vi "Update Bind RPC Template.vi"(8 "error in (no error)":errorcluster, 11 "Server Library (Library Item) in":refnum<vi>) -> (0 "error out":errorcluster, 3 "Server Library (Library Item) out":refnum<vi>)   [LabVIEW 2019, in "gRPC Scripting Tools.lvlib"]
uses:
  gRPC Scripting Tools.lvlib
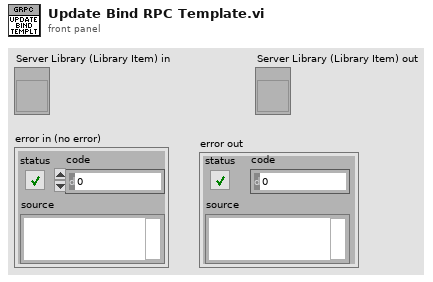
[diagram p1: front panel]
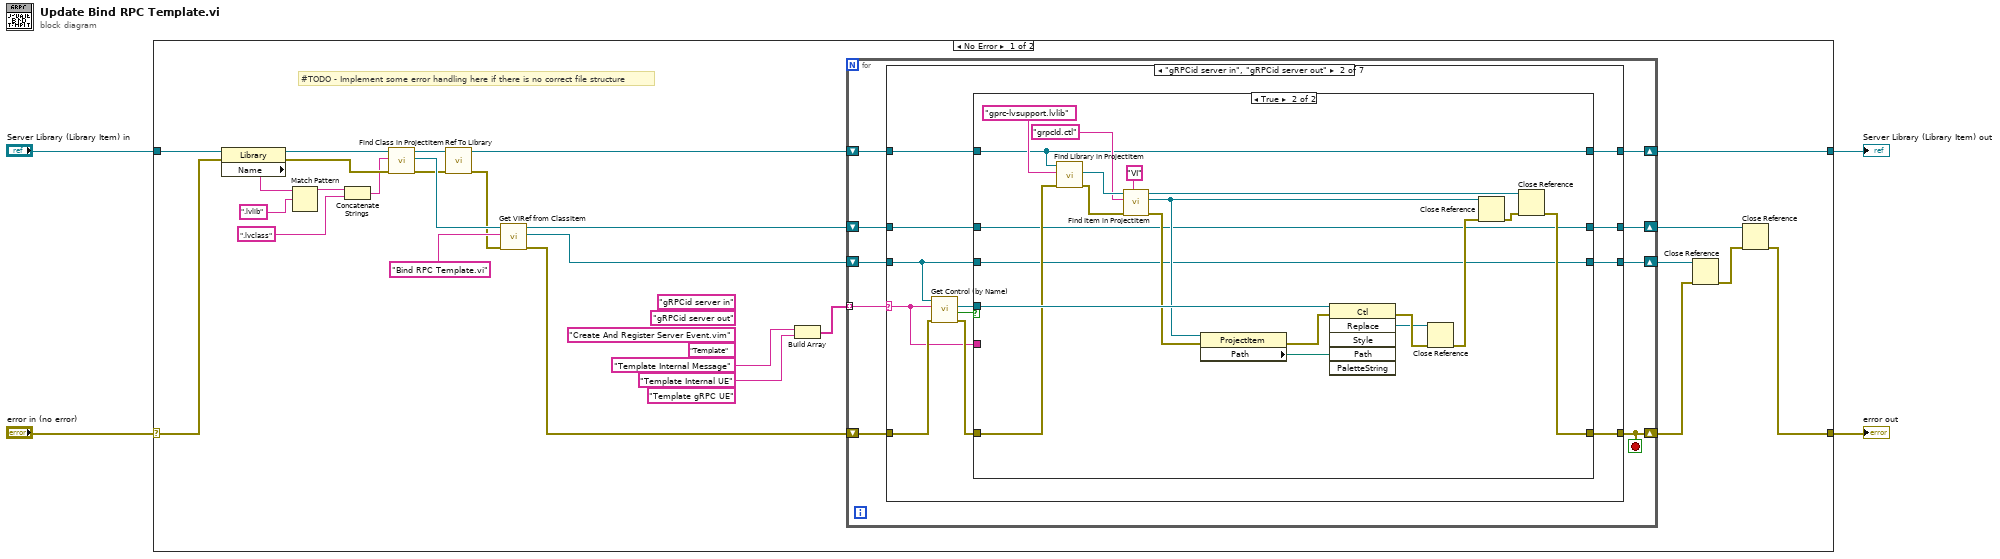
[diagram p0: block diagram]
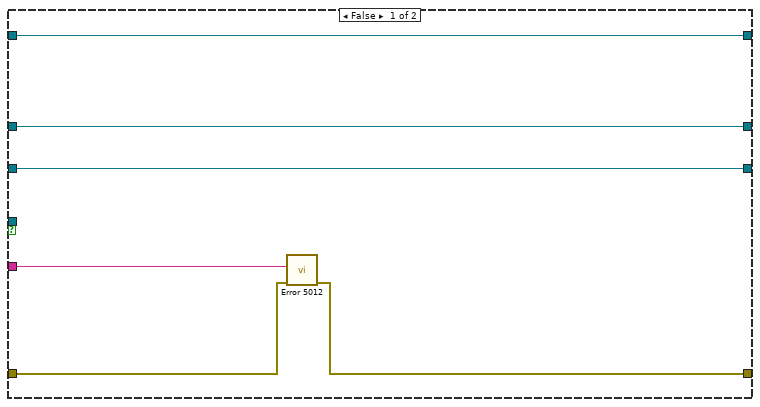
[diagram p3: hidden frame]
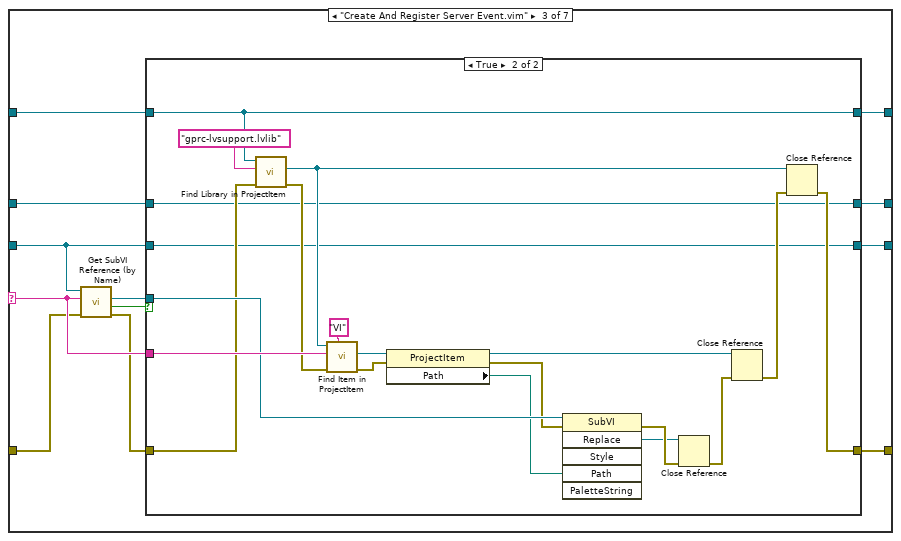
[diagram p4: hidden frame]
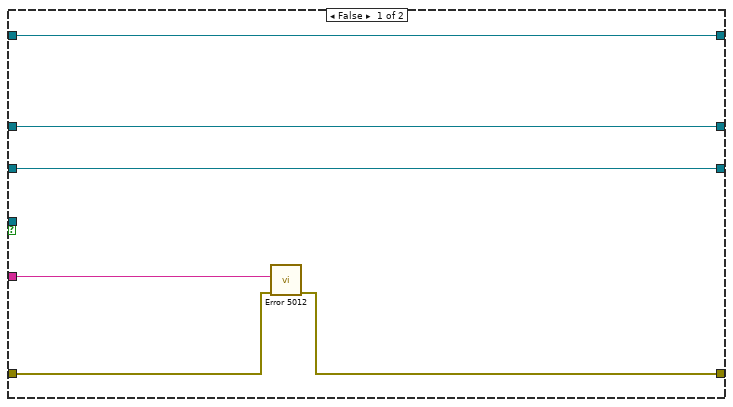
[diagram p5: hidden frame]
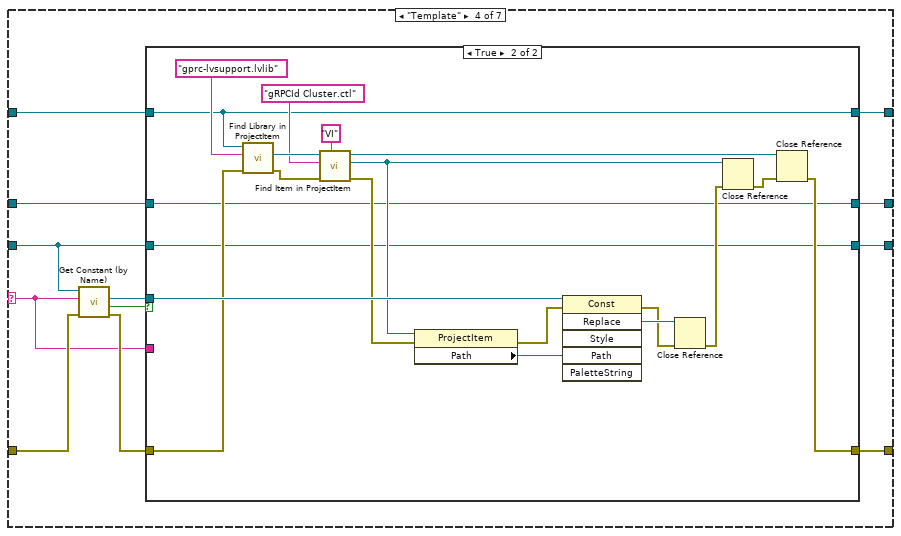
[diagram p6: hidden frame]
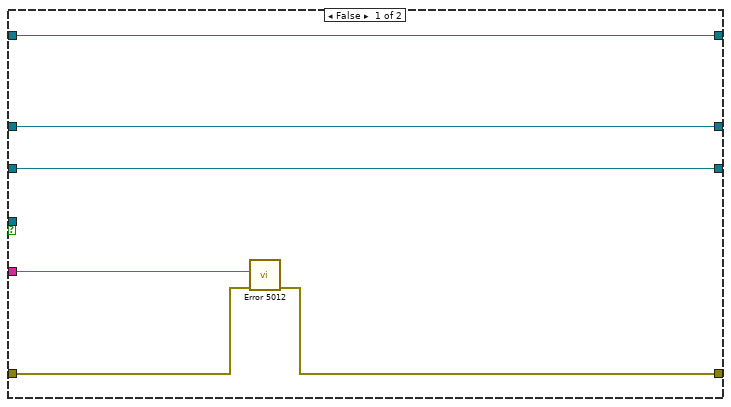
[diagram p7: hidden frame]
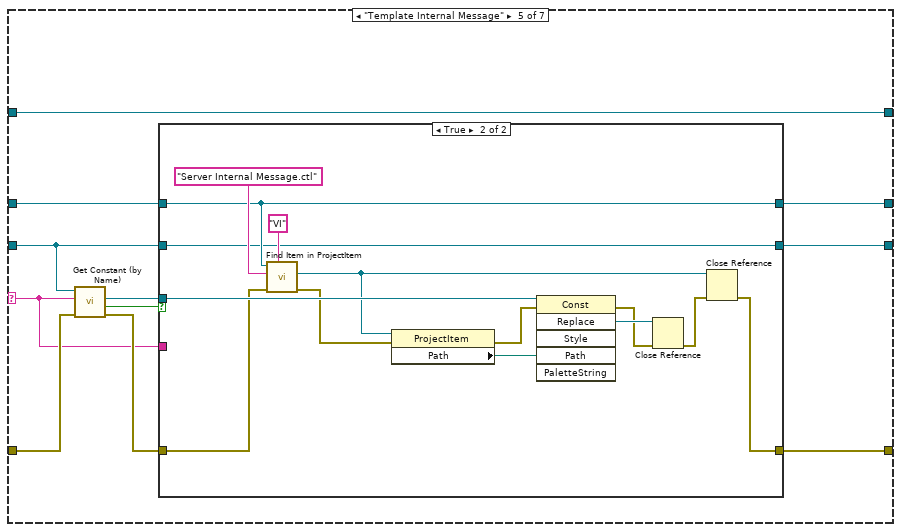
[diagram p8: hidden frame]
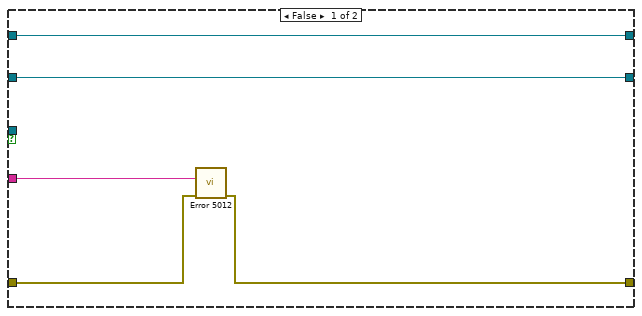
[diagram p9: hidden frame]
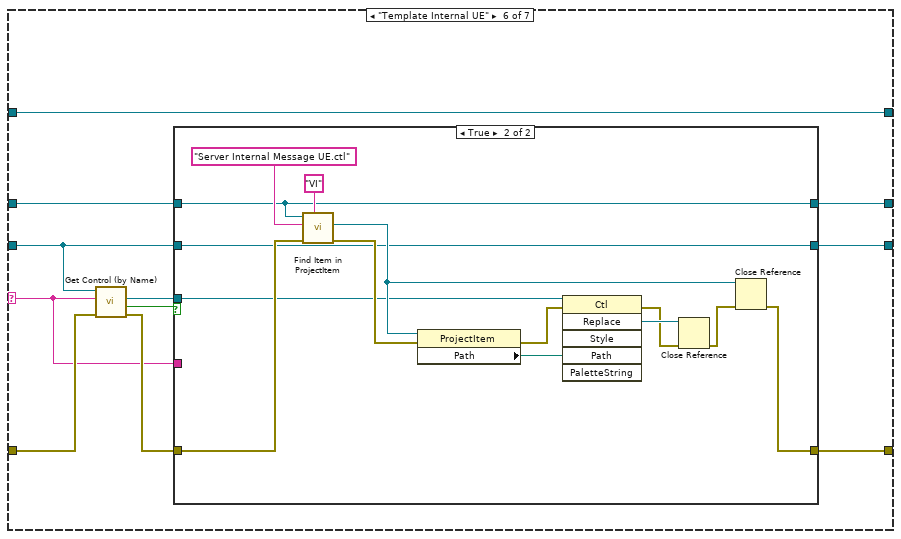
[diagram p10: hidden frame]
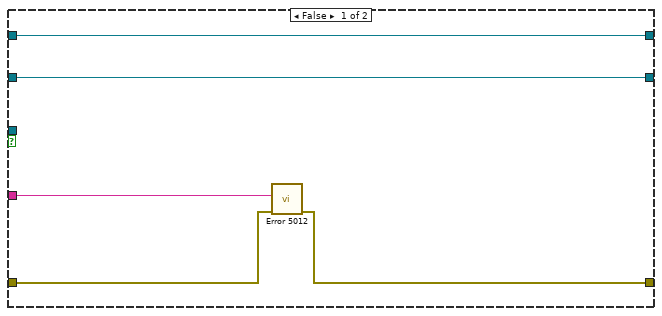
[diagram p11: hidden frame]
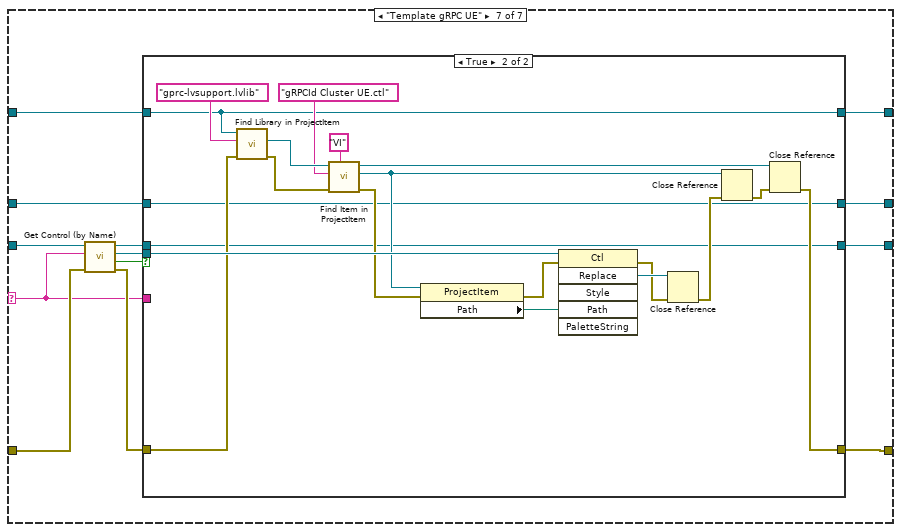
[diagram p12: hidden frame]
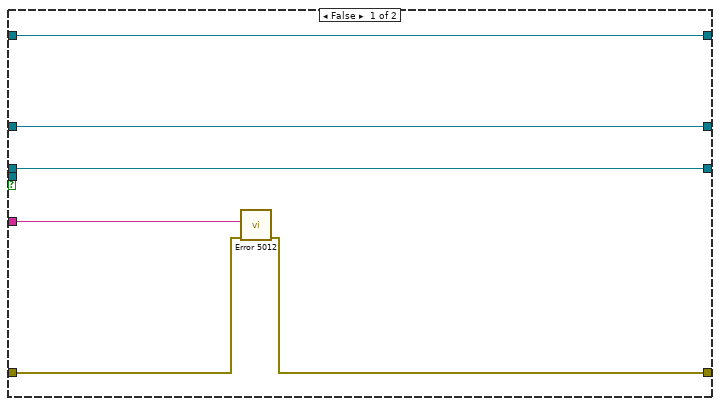
[diagram p13: hidden frame]
diagram:
  n1 = case shown="No Error" "error in (no error)" {
    selector: "error in (no error)" -> [w21 w259]
    tunnel: "Server Library (Library Item) in" -> [w29 w258]
    tunnel: [w8 w259] -> w3
    tunnel: [w10 w258] -> w1
    frame No Error {
      (unwired) "Template gRPC UE" ("Item Name")
      (unwired) "Template" ("Item Name")
      (unwired) "Create And Register Server Event.vim" ("Item Name")
      (unwired) "gRPCid server out" ("Item Name")
      (unwired) "gRPCid server in" ("Item Name")
      # "#TODO - Implement some error handling here if there is no correct file structure"
      n2 = property class="Library"(reference=w29, error in=w21) -> (reference out=w26:refnum<vi>, error out=w28:errorcluster, "Name"=w22:string)
      n3 = Match Pattern(string=w22, regular expression=".lvlib") -> (before substring=w24:string)  [unwired: 1 in, 3 out]
      n4 = Concatenate Strings(w24, ".lvclass" ("string")) -> (w27:string)
      n5 = call "Find Class in ProjectItem.vi"("error in (no error)"=w28, "Class Name"=w27, "ProjectItem in"=w26) -> ("error out"=w19:errorcluster, "LVClass out"=w31:refnum<vi>, "ProjectItem out"=w20:refnum<vi>)  [unwired: 5 in, 1 out]
      n6 = call "Ref To Library.vi"("error in (no error)"=w19, "ProjectItem in"=w20) -> ("error out"=w18:errorcluster, "Library out"=w15:refnum<vi>)  [unwired: 8 in]
      n7 = call "Get VIRef from ClassItem.vi"("error in (no error)"=w18, "Item Name"="Bind RPC Template.vi", "LVClassLibrary in"=w31) -> ("error out"=w12:errorcluster, "VIref out"=w11:refnum<vi>, "LVClassLibrary out"=w14:refnum<vi>)  [unwired: 5 in, 1 out]
      n8 = Build Array("Template Internal Message" ("Item Name"), "Template Internal UE" ("Item Name")) -> (w13:string[])
      n9 = for {
        shift-right: [w38] -> w10
        shift-left: w15 -> [w39]
        tunnel: w13 -> [w40] mode=indexing
        shift-right: [w32] -> w6
        shift-left: w12 -> [w37]
        shift-right: [w34] -> w9
        shift-left: w14 -> [w35]
        shift-right: [w33] -> w7
        shift-left: w11 -> [w36]
        stop <- w32 stop-if-true
        n10 = case shown="\"gRPCid server in\", \"gRPCid server out\"" w40 {
          selector: w40 -> [_ w45 w93 w121 w159 w189 w219]
          tunnel: w39 -> [w44 w56 w94 w132 w169 w199 w228]
          tunnel: [w44 w46 w83 w122 w169 w199 w224] -> w38
          tunnel: w36 -> [w41 w50 w87 w126 w161 w192 w231]
          tunnel: w37 -> [w43 w54 w91 w130 w167 w197 w230]
          tunnel: [w43 w52 w89 w128 w166 w198 w226] -> w32
          tunnel: w35 -> [w42 w48 w85 w124 w164 w194 w223]
          tunnel: [w42 w47 w84 w123 w162 w190 w222] -> w34
          tunnel: [w41 w49 w86 w125 w160 w191 w220] -> w33
          frame "None", Default {
          }
          frame "gRPCid server in", "gRPCid server out" {
            n11 = call "Get Control (by Name).vi"("error in (no error)"=w54, "Control Label"=w45, "Owner VI in"=w50) -> ("error out"=w53:errorcluster, "Found ?"=w51:bool, "Control Refnum"=w55:refnum<vi>)  [unwired: 5 in, 1 out]
            n12 = case shown="True" w51 {
              tunnel: w56 -> [w62 w63]
              tunnel: w55 -> [_ w78]
              tunnel: w53 -> [w59 w76]
              tunnel: [w57 w66] -> w52
              tunnel: w50 -> [w60 w65]
              tunnel: [w60 w65] -> w49
              tunnel: w48 -> [w61 w64]
              tunnel: [w61 w64] -> w47
              tunnel: [w62 w63] -> w46
              tunnel: w45 -> [w58 _]
              frame False {
                n13 = call "Error 5012.vi"("error in (no error)"=w59, "Element Name"=w58) -> ("error out"=w57:errorcluster)  [unwired: 9 in]
              }
              frame True {
                n14 = call "Find Library in ProjectItem.vi"("error in (no error)"=w76, "Library Name"="gprc-lvsupport.lvlib", "ProjectItem in"=w63) -> ("error out"=w75:errorcluster, "Library out"=w81:refnum<vi>)  [unwired: 5 in, 2 out]
                n15 = call "Find Item in ProjectItem.vi"("Item Type"="VI", "error in (no error)"=w75, "Name"="grpcId.ctl", "ProjectItem in"=w81) -> ("error out"=w74:errorcluster, "Item Refnum out"=w69:refnum<vi>, "ProjectItem out"=w67:refnum<vi>)  [unwired: 4 in, 1 out]
                n16 = property class="ProjectItem"(reference=w69, error in=w74) -> (error out=w71:errorcluster, "Path"=w77:path)  [unwired: 1 out]
                n17 = invoke class="Ctl" method="Replace"(reference=w78, error in=w71, "Path"=w77) -> (error out=w73:errorcluster, "Replace"=w72:refnum<vi>)  [unwired: 3 in, 4 out]
                n18 = Close Reference(reference=w72, error in (no error)=w73) -> (error out=w70:errorcluster)
                n19 = Close Reference(reference=w69, error in (no error)=w70) -> (error out=w68:errorcluster)
                n20 = Close Reference(reference=w67, error in (no error)=w68) -> (error out=w66:errorcluster)
              }
            }
          }
          frame "Create And Register Server Event.vim" {
            n21 = call "Get SubVI Reference (by Name).vi"("error in (no error)"=w91, "SubVI Name"=w93, "Owner VI in"=w87) -> ("error out"=w90:errorcluster, "Found ?"=w88:bool, "SubVI Refnum out"=w92:refnum<vi>)  [unwired: 5 in, 1 out]
            n22 = case shown="True" w88 {
              tunnel: w94 -> [w100 w101]
              tunnel: w93 -> [w96 w118]
              tunnel: w92 -> [_ w117]
              tunnel: w90 -> [w97 w112]
              tunnel: [w95 w104] -> w89
              tunnel: w87 -> [w98 w103]
              tunnel: [w98 w103] -> w86
              tunnel: w85 -> [w99 w102]
              tunnel: [w99 w102] -> w84
              tunnel: [w100 w101] -> w83
              frame False {
                n23 = call "Error 5012.vi"("error in (no error)"=w97, "Element Name"=w96) -> ("error out"=w95:errorcluster)  [unwired: 9 in]
              }
              frame True {
                n24 = call "Find Library in ProjectItem.vi"("error in (no error)"=w112, "Library Name"="gprc-lvsupport.lvlib", "ProjectItem in"=w101) -> ("error out"=w111:errorcluster, "Library out"=w106:refnum<vi>)  [unwired: 5 in, 2 out]
                n25 = call "Find Item in ProjectItem.vi"("Item Type"="VI", "error in (no error)"=w111, "Name"=w118, "ProjectItem in"=w106) -> ("error out"=w110:errorcluster, "Item Refnum out"=w116:refnum<vi>)  [unwired: 4 in, 2 out]
                n26 = property class="ProjectItem"(reference=w116, error in=w110) -> (reference out=w108:refnum<vi>, error out=w109:errorcluster, "Path"=w115:path)
                n27 = invoke class="SubVI" method="Replace"(reference=w117, error in=w109, "Path"=w115) -> (error out=w114:errorcluster, "Replace"=w113:refnum<vi>)  [unwired: 3 in, 4 out]
                n28 = Close Reference(reference=w113, error in (no error)=w114) -> (error out=w107:errorcluster)
                n29 = Close Reference(reference=w108, error in (no error)=w107) -> (error out=w105:errorcluster)
                n30 = Close Reference(reference=w106, error in (no error)=w105) -> (error out=w104:errorcluster)
              }
            }
          }
          frame "Template" {
            n31 = call "Get Constant (by Name).vi"("error in (no error)"=w130, "Constant Label"=w121, "Owner VI in"=w126) -> ("error out"=w129:errorcluster, "Found ?"=w127:bool, "Const ref out"=w131:refnum<vi>)  [unwired: 5 in, 1 out]
            n32 = case shown="True" w127 {
              tunnel: w132 -> [w138 w139]
              tunnel: w131 -> [_ w152]
              tunnel: w129 -> [w134 w145]
              tunnel: [w133 w142] -> w128
              tunnel: w126 -> [w136 w141]
              tunnel: [w136 w141] -> w125
              tunnel: w124 -> [w137 w140]
              tunnel: [w137 w140] -> w123
              tunnel: [w138 w139] -> w122
              tunnel: w121 -> [w135 _]
              frame False {
                n33 = call "Error 5012.vi"("error in (no error)"=w134, "Element Name"=w135) -> ("error out"=w133:errorcluster)  [unwired: 9 in]
              }
              frame True {
                n34 = call "Find Library in ProjectItem.vi"("error in (no error)"=w145, "Library Name"="gprc-lvsupport.lvlib", "ProjectItem in"=w139) -> ("error out"=w144:errorcluster, "Library out"=w157:refnum<vi>)  [unwired: 5 in, 2 out]
                n35 = call "Find Item in ProjectItem.vi"("Item Type"="VI", "error in (no error)"=w144, "Name"="gRPCId Cluster.ctl", "ProjectItem in"=w157) -> ("error out"=w143:errorcluster, "Item Refnum out"=w149:refnum<vi>, "ProjectItem out"=w147:refnum<vi>)  [unwired: 4 in, 1 out]
                n36 = property class="ProjectItem"(reference=w149, error in=w143) -> (error out=w153:errorcluster, "Path"=w154:path)  [unwired: 1 out]
                n37 = invoke class="Const" method="Replace"(reference=w152, error in=w153, "Path"=w154) -> (error out=w150:errorcluster, "Replace"=w151:refnum<vi>)  [unwired: 3 in, 4 out]
                n38 = Close Reference(reference=w151, error in (no error)=w150) -> (error out=w148:errorcluster)
                n39 = Close Reference(reference=w149, error in (no error)=w148) -> (error out=w146:errorcluster)
                n40 = Close Reference(reference=w147, error in (no error)=w146) -> (error out=w142:errorcluster)
              }
            }
          }
          frame "Template Internal Message" {
            n41 = call "Get Constant (by Name).vi"("error in (no error)"=w167, "Constant Label"=w159, "Owner VI in"=w161) -> ("error out"=w165:errorcluster, "Found ?"=w163:bool, "Const ref out"=w168:refnum<vi>)  [unwired: 5 in, 1 out]
            n42 = case shown="True" w163 {
              tunnel: w168 -> [_ w184]
              tunnel: [w170 w178] -> w166
              tunnel: w165 -> [w171 w177]
              tunnel: w164 -> [w174 w176]
              tunnel: [w174 w176] -> w162
              tunnel: w161 -> [w173 w175]
              tunnel: [w173 w175] -> w160
              tunnel: w159 -> [w172 _]
              frame False {
                n43 = call "Error 5012.vi"("error in (no error)"=w171, "Element Name"=w172) -> ("error out"=w170:errorcluster)  [unwired: 9 in]
              }
              frame True {
                n44 = call "Find Item in ProjectItem.vi"("Item Type"="VI", "error in (no error)"=w177, "Name"="Server Internal Message.ctl", "ProjectItem in"=w176) -> ("error out"=w179:errorcluster, "Item Refnum out"=w181:refnum<vi>)  [unwired: 4 in, 2 out]
                n45 = property class="ProjectItem"(reference=w181, error in=w179) -> (error out=w185:errorcluster, "Path"=w186:path)  [unwired: 1 out]
                n46 = invoke class="Const" method="Replace"(reference=w184, error in=w185, "Path"=w186) -> (error out=w182:errorcluster, "Replace"=w183:refnum<vi>)  [unwired: 3 in, 4 out]
                n47 = Close Reference(reference=w183, error in (no error)=w182) -> (error out=w180:errorcluster)
                n48 = Close Reference(reference=w181, error in (no error)=w180) -> (error out=w178:errorcluster)
              }
            }
          }
          frame "Template Internal UE" {
            n49 = call "Get Control (by Name).vi"("error in (no error)"=w197, "Control Label"=w189, "Owner VI in"=w192) -> ("error out"=w196:errorcluster, "Found ?"=w193:bool, "Control Refnum"=w195:refnum<vi>)  [unwired: 5 in, 1 out]
            n50 = case shown="True" w193 {
              tunnel: [w201 w209] -> w198
              tunnel: w196 -> [w202 w208]
              tunnel: w195 -> [_ w207]
              tunnel: w194 -> [w204 w205]
              tunnel: w192 -> [w203 w206]
              tunnel: [w203 w206] -> w191
              tunnel: [w204 w205] -> w190
              tunnel: w189 -> [w200 _]
              frame False {
                n51 = call "Error 5012.vi"("error in (no error)"=w202, "Element Name"=w200) -> ("error out"=w201:errorcluster)  [unwired: 9 in]
              }
              frame True {
                n52 = call "Find Item in ProjectItem.vi"("Item Type"="VI", "error in (no error)"=w208, "Name"="Server Internal Message UE.ctl", "ProjectItem in"=w205) -> ("error out"=w210:errorcluster, "Item Refnum out"=w212:refnum<vi>)  [unwired: 4 in, 2 out]
                n53 = property class="ProjectItem"(reference=w212, error in=w210) -> (error out=w215:errorcluster, "Path"=w216:path)  [unwired: 1 out]
                n54 = invoke class="Ctl" method="Replace"(reference=w207, error in=w215, "Path"=w216) -> (error out=w213:errorcluster, "Replace"=w214:refnum<vi>)  [unwired: 3 in, 4 out]
                n55 = Close Reference(reference=w214, error in (no error)=w213) -> (error out=w211:errorcluster)
                n56 = Close Reference(reference=w212, error in (no error)=w211) -> (error out=w209:errorcluster)
              }
            }
          }
          frame "Template gRPC UE" {
            n57 = call "Get Control (by Name).vi"("error in (no error)"=w230, "Control Label"=w219, "Owner VI in"=w231) -> ("error out"=w227:errorcluster, "Found ?"=w225:bool, "Control Refnum"=w229:refnum<vi>, "Owner VI out"=w221:refnum<vi>)  [unwired: 5 in]
            n58 = case shown="True" w225 {
              tunnel: w229 -> [_ w252]
              tunnel: w228 -> [w237 w240]
              tunnel: w227 -> [w234 w246]
              tunnel: [w232 w241] -> w226
              tunnel: [w237 w240] -> w224
              tunnel: w223 -> [w236 w239]
              tunnel: [w236 w239] -> w222
              tunnel: w221 -> [w235 w238]
              tunnel: [w235 w238] -> w220
              tunnel: w219 -> [w233 _]
              frame False {
                n59 = call "Error 5012.vi"("error in (no error)"=w234, "Element Name"=w233) -> ("error out"=w232:errorcluster)  [unwired: 9 in]
              }
              frame True {
                n60 = call "Find Library in ProjectItem.vi"("error in (no error)"=w246, "Library Name"="gprc-lvsupport.lvlib", "ProjectItem in"=w240) -> ("error out"=w247:errorcluster, "Library out"=w250:refnum<vi>)  [unwired: 5 in, 2 out]
                n61 = call "Find Item in ProjectItem.vi"("Item Type"="VI", "error in (no error)"=w247, "Name"="gRPCId Cluster UE.ctl", "ProjectItem in"=w250) -> ("error out"=w245:errorcluster, "Item Refnum out"=w244:refnum<vi>, "ProjectItem out"=w243:refnum<vi>)  [unwired: 4 in, 1 out]
                n62 = property class="ProjectItem"(reference=w244, error in=w245) -> (error out=w256:errorcluster, "Path"=w257:path)  [unwired: 1 out]
                n63 = invoke class="Ctl" method="Replace"(reference=w252, error in=w256, "Path"=w257) -> (error out=w254:errorcluster, "Replace"=w255:refnum<vi>)  [unwired: 3 in, 4 out]
                n64 = Close Reference(reference=w255, error in (no error)=w254) -> (error out=w253:errorcluster)
                n65 = Close Reference(reference=w244, error in (no error)=w253) -> (error out=w242:errorcluster)
                n66 = Close Reference(reference=w243, error in (no error)=w242) -> (error out=w241:errorcluster)
              }
            }
          }
        }
      }
      n67 = Close Reference(reference=w7, error in (no error)=w6) -> (error out=w5:errorcluster)
      n68 = Close Reference(reference=w9, error in (no error)=w5) -> (error out=w8:errorcluster)
    }
    frame Error {
    }
  }
  "error out" <- w3
  "Server Library (Library Item) out" <- w1
